vi "DOA_to_phase calc.vi"(10 "f set (Hz)":dbl[](array[numeric]), 11 "DOA (deg)":dbl) -> (3 "phase":ext[][](array[numeric]))   [LabVIEW 2022 SP3]
uses:
  <vilib>/Analysis/1siggen.llb/Ramp Pattern by Samples.vi
  <vilib>/Analysis/NI_AALBase.lvlib
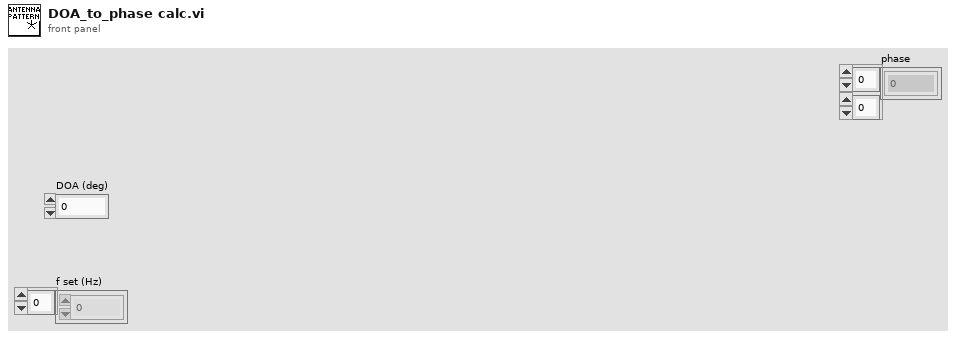
[diagram p1: front panel]
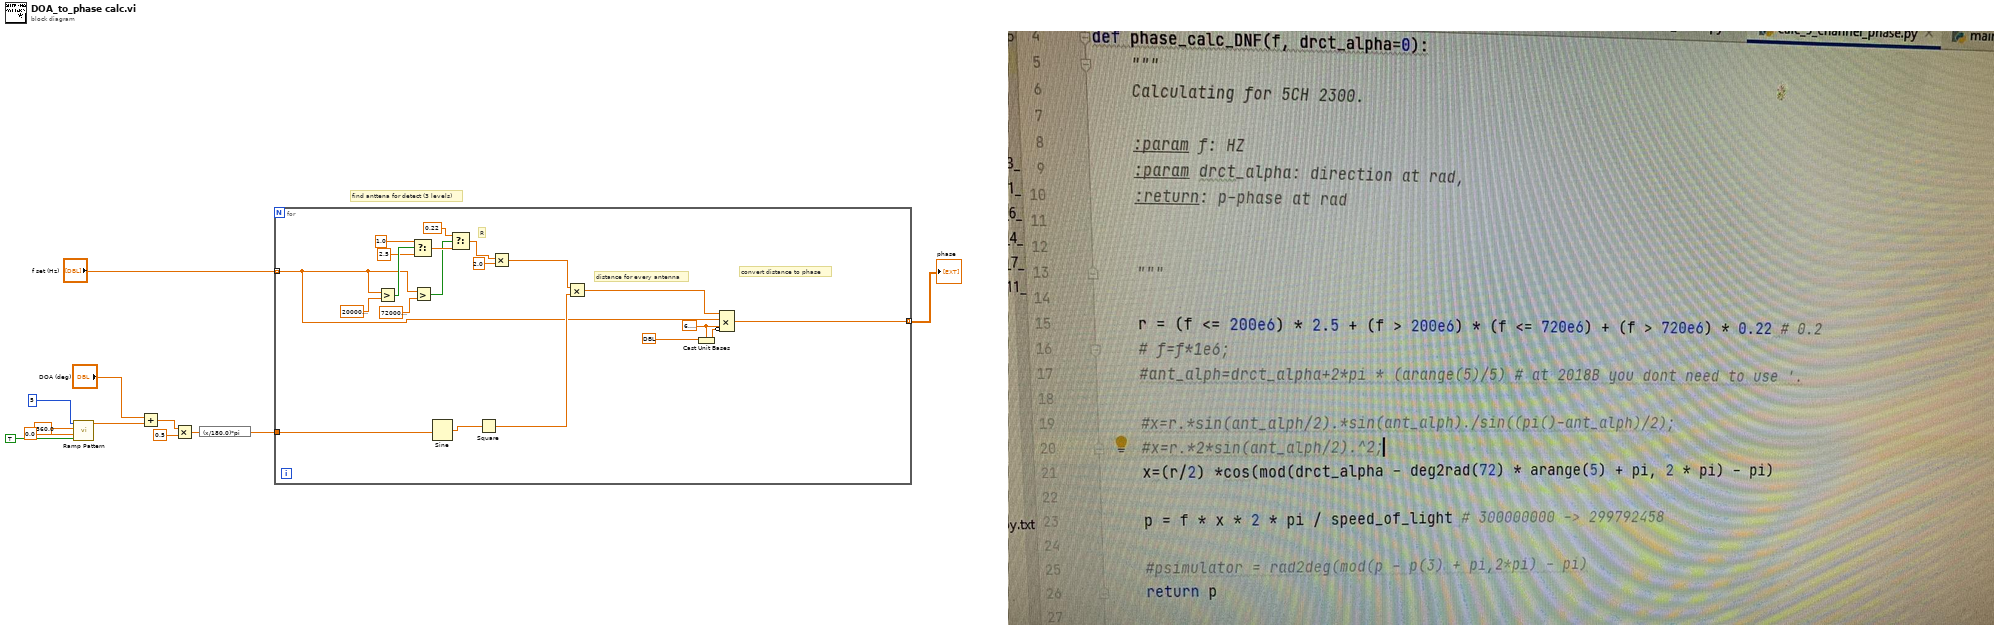
[diagram p0: block diagram]
diagram:
  # "find anttena for detect (3 levels)"
  n1 = call-poly <vilib>:"Ramp Pattern.vi"("exclude end?"=TRUE, "start"=0.0, "end"=360.0, "samples"=5) -> ("Ramp Pattern"=w6:dbl[])  [unwired: 6 in, 1 out]
  n2 = Add(x="DOA (deg)", y=w6) -> (x+y=w4:dbl[])
  n3 = Multiply(x=w4, y=0.5) -> (x*y=w3:dbl[])
  n4 = expression code="(x/180.0)*pi" ("degrees to radians")(w3) -> (w2:dbl[])
  n5 = for {
    tunnel: "f set (Hz)" -> [w17] mode=indexing
    tunnel: w2 -> [w22]
    tunnel: [w16] -> w1 mode=indexing
    w14 = 6.283185307179586
    # "convert distance to phase"
    # "distance for every antenna"
    # "R"
    n6 = Greater?(x=w17, y=200000000.0) -> (0:w30:bool)
    n7 = Select(t=1.0, s=w30, f=2.5) -> (s? t:f=w29:dbl)
    n8 = Greater?(x=w17, y=720000000.0) -> (0:w25:bool)
    n9 = Sine(x=w22) -> (sin(x)=w21:dbl[])
    n10 = Select(t=0.22, s=w25, f=w29) -> (s? t:f=w23:dbl)
    n11 = Square(x=w21) -> (x^2=w19:dbl[])
    n12 = Multiply(x=w23, y=2.0) -> (x*y=w20:dbl)
    n13 = Multiply(x=w20, y=w19) -> (x*y=w18:dbl[])
    n14 = Cast Unit Bases(0:ext[unit] 299792458.0, 1:w14) -> (2:w13:ext)
    n15 = Compound Arithmetic op=MULTIPLY(w18, w17, w14, invert w13) -> (w16:ext[])
  }
  "phase" <- w1
